vi "Get Front Panel Reference.vi"(8 "error in (no error)":errorcluster, 11 "CIF_UI in":refnum<class "CIF_UI.lvclass">) -> (0 "error out":errorcluster, 3 "CIF_UI out":refnum<class "CIF_UI.lvclass">)   [LabVIEW 2021, in "CIF_UI.lvclass"]
uses:
  CIF_UI.lvclass
  CIF_UI.lvclass/CIF_UI.ctl
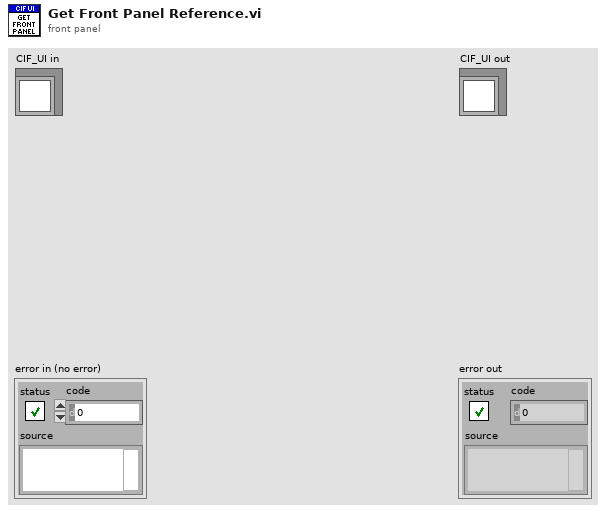
[diagram p1: front panel]
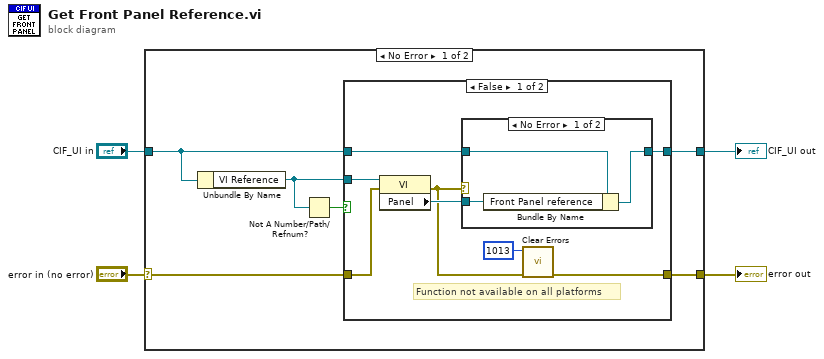
[diagram p0: block diagram]
diagram:
  n1 = case shown="No Error" "error in (no error)" {
    selector: "error in (no error)" -> [w10 w26]
    tunnel: [w5 w26] -> w3
    tunnel: [w8 w25] -> w1
    tunnel: "CIF_UI in" -> [w9 w25]
    frame No Error {
      n2 = Unbundle By Name(w9) -> ("VI Reference"=w7:refnum<vi>)
      n3 = Not A Number/Path/Refnum?(number/path/refnum=w7) -> (NaN/Path/Refnum?=w6:bool)
      n4 = case shown="False" w6 {
        tunnel: w10 -> [w11 w24]
        tunnel: w9 -> [w18 w23]
        tunnel: [w17 w23] -> w8
        tunnel: w7 -> [w14 _]
        tunnel: [w12 w24] -> w5
        frame False {
          # "Function not available on all platforms"
          n5 = property class="VI"(reference=w14, error in=w11) -> (error out=w15:errorcluster, "Panel"=w16:refnum<vi>)  [unwired: 1 out]
          n6 = case shown="No Error" w15 {
            tunnel: w18 -> [w21 w22]
            tunnel: [w19 w22] -> w17
            tunnel: w16 -> [w20 _]
            frame No Error {
              n7 = Bundle By Name(cluster=w21, "Front Panel reference"=w20) -> (w19:refnum<class "CIF_UI.lvclass">)
            }
            frame Error {
            }
          }
          n8 = call <vilib>:"Clear Errors.vi"("error in (no error)"=w15, "specific error code to clear (0: all)"=1013) -> ("error out"=w12:errorcluster)  [unwired: 4 in, 1 out]
        }
        frame True {
          # "VI Reference is not valid"
        }
      }
    }
    frame Error {
    }
  }
  "error out" <- w3
  "CIF_UI out" <- w1
